vi "Teleop_System_Acquire_Decide.vi"(8 "error in (no error)":errorcluster) -> (0 "error out":errorcluster)   [LabVIEW 2019]
uses:
  <vilib>/Rock Robotics/WPI/Joystick/WPI_JoystickArcadeMapping.vi
  <vilib>/Rock Robotics/WPI/ThirdParty/JAS_Junk/TrajLib/Trajectory_Library.lvlib
  Teleop_System_Globals.vi
  <vilib>/Rock Robotics/WPI/Joystick/XBox Buttons Indexer.ctl
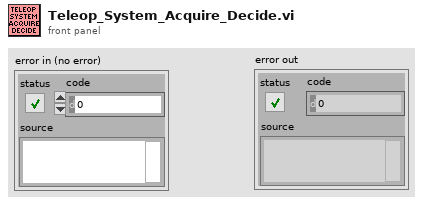
[diagram p1: front panel]
types:
  T1 = typedef "XBox Buttons Indexer.ctl" = enum16{"A", "B", "X", "Y", "Left Bumper", "Right Bumper", "Back", "Start", "Left Joystick", "Right Joystick"}
  T2 = typedef "WPI_JoystickDevRef.ctl" = cluster{"Device":T3}
  T3 = typedef "WPI_JoystickDeviceEnum.ctl" = enum16{"USB 0", "USB 1", "USB 2", "USB 3", "USB 4", "USB 5"}
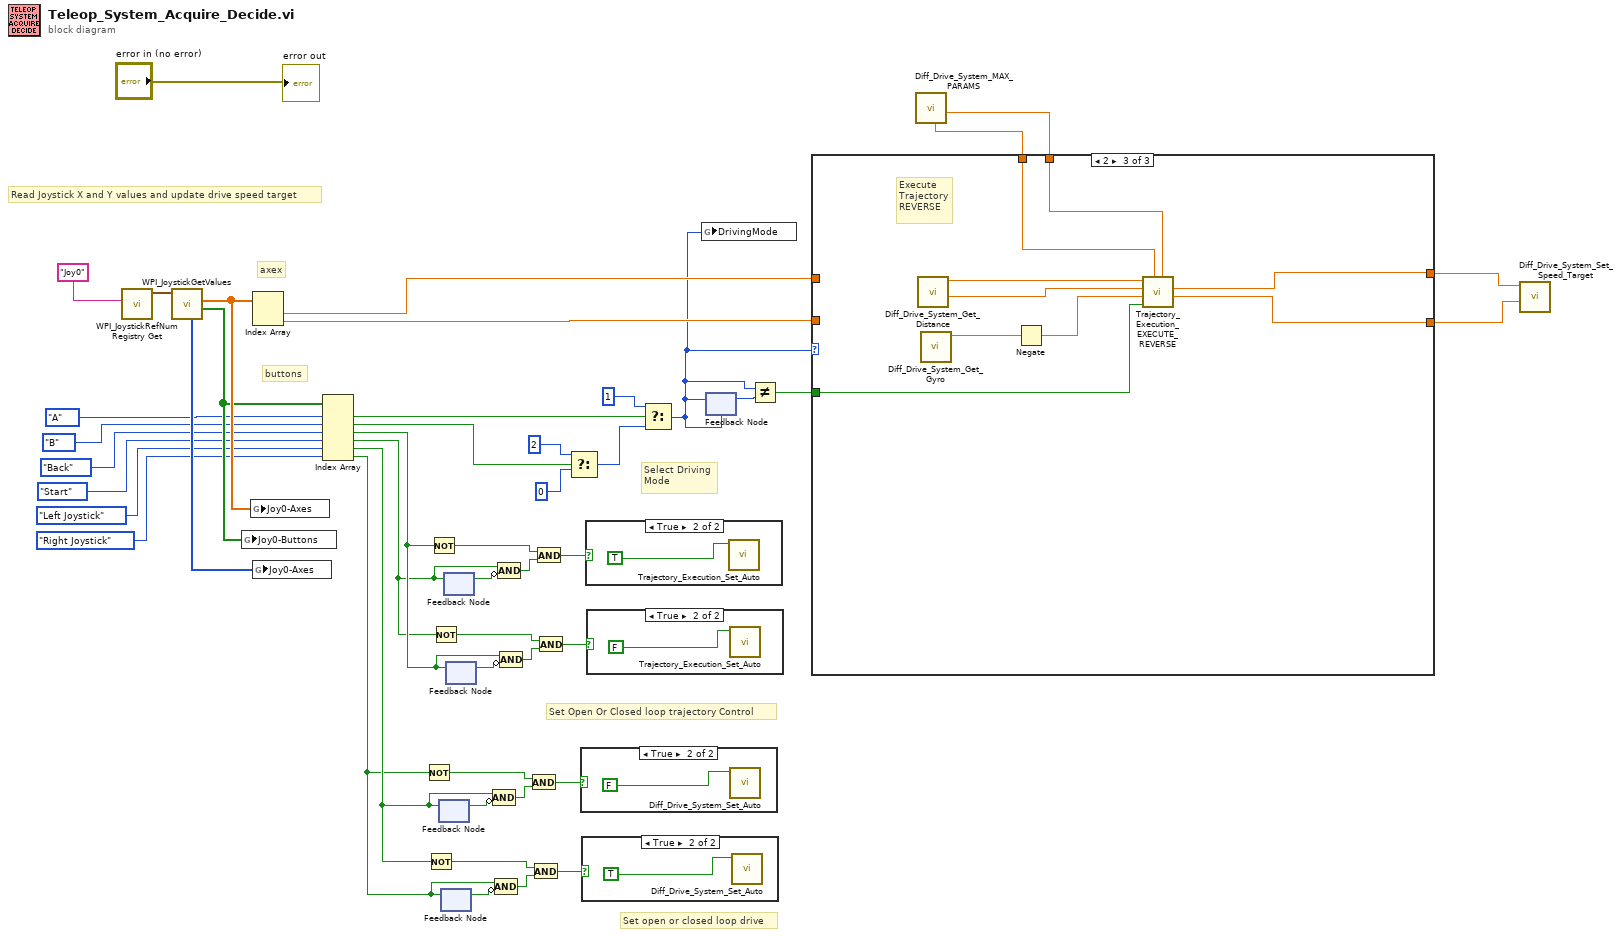
[diagram p0: block diagram]
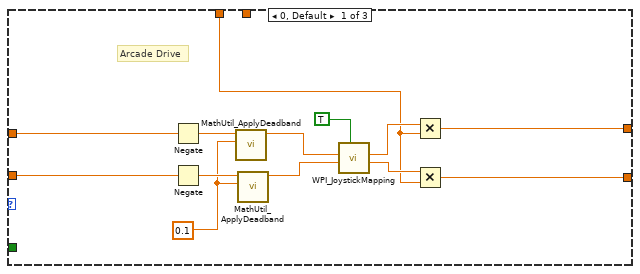
[diagram p6: hidden frame]
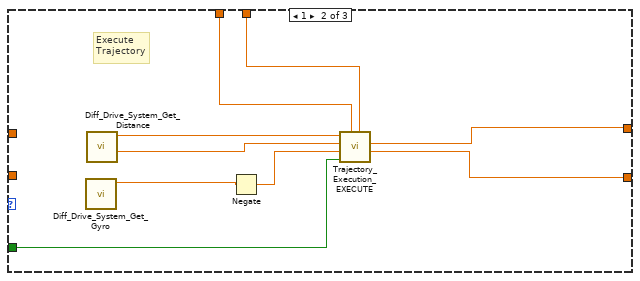
[diagram p7: hidden frame]
diagram:
  # "Set open or closed loop drive"
  # "Set Open Or Closed loop trajectory Control"
  # "Select Driving\nMode"
  # "buttons"
  # "axex"
  # "Read Joystick X and Y values and update drive speed target"
  n1 = call <vilib>:"WPI_JoystickRefNum Registry Get.vi"("refnum name"="Joy0") -> ("JoystickDevRef"=w28:T2)  [unwired: 1 in, 9 out]
  n2 = call <vilib>:"WPI_JoystickGetValues.vi"("JoystickDevRef"=w28) -> ("Buttons"=w25:bool[], "Axes"=w26:dbl[], "POVs"=w24:i16[])  [unwired: 6 in, 2 out]
  n3 = global write "Teleop_System_Globals.vi" "Joy0-Buttons"(w25) -> ()
  n4 = global write "Teleop_System_Globals.vi" "Joy0-Axes"(w26) -> ()
  n5 = Index Array(array=w26) -> (element #1=w29:dbl, element #2=w30:dbl)  [unwired: 2 in]
  n6 = global write "Teleop_System_Globals.vi" "Joy0-Axes"(w24) -> ()
  n7 = Index Array(array=w25, index #1=XBox_Buttons_Indexer."A" ("XBox Buttons"), index #2=XBox_Buttons_Indexer."B" ("XBox Buttons"), index #3=XBox_Buttons_Indexer."Back" ("XBox Buttons"), index #4=XBox_Buttons_Indexer."Start" ("XBox Buttons"), index #5=XBox_Buttons_Indexer."Left Joystick" ("XBox Buttons"), index #6=XBox_Buttons_Indexer."Right Joystick" ("XBox Buttons")) -> (element #1=w32:bool, element #2=w38:bool, element #3=w9:bool, element #4=w8:bool, element #5=w3:bool, element #6=w2:bool)
  n8 = Not(x=w2) -> (.not. x?=w14:bool)
  n9 = Not(x=w3) -> (.not. x?=w17:bool)
  n10 = Not(x=w9) -> (.not. x?=w42:bool)
  n11 = Not(x=w8) -> (.not. x?=w45:bool)
  n12 = feedback #1() -> (w12:bool)  [unwired: 1 in]
  n13 = feedback-in #1(w3) -> ()
  n14 = feedback #2() -> (w15:bool)  [unwired: 1 in]
  n15 = feedback-in #2(w2) -> ()
  n16 = feedback #3() -> (w40:bool)  [unwired: 1 in]
  n17 = feedback-in #3(w8) -> ()
  n18 = feedback #4() -> (w43:bool)  [unwired: 1 in]
  n19 = feedback-in #4(w9) -> ()
  n20 = Compound Arithmetic op=AND(w3, invert w12) -> (w13:bool)
  n21 = Compound Arithmetic op=AND(w2, invert w15) -> (w16:bool)
  n22 = Compound Arithmetic op=AND(w8, invert w40) -> (w41:bool)
  n23 = Compound Arithmetic op=AND(w9, invert w43) -> (w44:bool)
  n24 = And(x=w14, y=w13) -> (x .and. y?=w19:bool)
  n25 = And(x=w17, y=w16) -> (x .and. y?=w18:bool)
  n26 = And(x=w42, y=w41) -> (x .and. y?=w47:bool)
  n27 = And(x=w45, y=w44) -> (x .and. y?=w46:bool)
  n28 = Select(t=2, s=w38, f=0) -> (s? t:f=w37:i32)
  n29 = case shown="True" w19 {
    frame False {
    }
    frame True {
      n30 = call "Diff_Drive_System_Set_Auto.vi"("Auto Mode"=FALSE ("Traj_RamseteEnabled")) -> ()  [unwired: 11 in]
    }
  }
  n31 = case shown="True" w18 {
    frame False {
    }
    frame True {
      n32 = call "Diff_Drive_System_Set_Auto.vi"("Auto Mode"=TRUE ("Traj_RamseteEnabled")) -> ()  [unwired: 11 in]
    }
  }
  n33 = case shown="True" w47 {
    frame False {
    }
    frame True {
      n34 = call "Trajectory_Execution_Set_Auto.vi"("Ramsete AUTO"=TRUE ("Traj_RamseteEnabled")) -> ()  [unwired: 11 in]
    }
  }
  n35 = case shown="True" w46 {
    frame False {
    }
    frame True {
      n36 = call "Trajectory_Execution_Set_Auto.vi"("Ramsete AUTO"=FALSE ("Traj_RamseteEnabled")) -> ()  [unwired: 11 in]
    }
  }
  n37 = Select(t=1, s=w32, f=w37) -> (s? t:f=w20:i32)
  n38 = global write "Teleop_System_Globals.vi" "DrivingMode"(w20) -> ()
  n39 = feedback #5(w20) -> (w33:i32)
  n40 = feedback-in #5(w20) -> ()
  n41 = Not Equal?(x=w20, y=w33) -> (x != y?=w34:bool)
  n42 = call "Diff_Drive_System_MAX_PARAMS.vi"() -> ("Effective TrackWidth Ft"=w39:dbl, "Max Drive Speed Ft/Sec"=w1:dbl)  [unwired: 9 in, 1 out]
  n43 = case shown="2" w20 {
    tunnel: w29 -> [w63 _ _]
    tunnel: w30 -> [w62 _ _]
    tunnel: [w61 w70 w79] -> w22
    tunnel: [w60 w69 w78] -> w21
    tunnel: w1 -> [w57 w71 w80]
    tunnel: w34 -> [_ w73 w82]
    tunnel: w39 -> [_ w68 w77]
    frame 0, Default {
      w52 = 0.1 ("Deadband")
      # "Arcade Drive"
      n44 = Negate(x=w63) -> (-x=w55:dbl)
      n45 = Negate(x=w62) -> (-x=w54:dbl)
      n46 = call <vilib>:"MathUtil_ApplyDeadband.vi"("Deadband"=w52, "Value"=w55) -> ("Result"=w56:dbl)  [unwired: 9 in]
      n47 = call <vilib>:"MathUtil_ApplyDeadband.vi"("Deadband"=w52, "Value"=w54) -> ("Result"=w53:dbl)  [unwired: 9 in]
      n48 = call-poly <vilib>:"WPI_JoystickMapping.vi"("Square Inputs"=TRUE, "Y axis value"=w53, "X axis value"=w56) -> ("Right Motor Value"=w58:dbl, "Left Motor Value"=w59:dbl)  [unwired: 7 in]
      n49 = Multiply(x=w59, y=w57) -> (x*y=w61:dbl)
      n50 = Multiply(x=w58, y=w57) -> (x*y=w60:dbl)
    }
    frame 1 {
      # "Execute\nTrajectory"
      n51 = call "Diff_Drive_System_Get_Gyro.vi"() -> ("Gyro_DEG"=w67:dbl)  [unwired: 10 in, 1 out]
      n52 = call "Diff_Drive_System_Get_Distance.vi"() -> ("Right Distance FT"=w65:dbl, "Left Distance FT"=w66:dbl)  [unwired: 10 in]
      n53 = Negate(x=w67) -> (-x=w72:dbl)
      n54 = call "Trajectory_Execution_EXECUTE.vi"("Track Width FT"=w68, "Max Speed\nFT/SEC"=w71, "Init"=w73, "Gyro Continous\n (inc counterclockwise)"=w72, "Right Distance"=w65, "Left Distance"=w66) -> ("Right Speed Target"=w69:dbl, "Left Speed Target"=w70:dbl)  [unwired: 1 in, 3 out]
    }
    frame 2 {
      # "Execute\nTrajectory\nREVERSE"
      n55 = call "Diff_Drive_System_Get_Distance.vi"() -> ("Right Distance FT"=w74:dbl, "Left Distance FT"=w75:dbl)  [unwired: 10 in]
      n56 = call "Diff_Drive_System_Get_Gyro.vi"() -> ("Gyro_DEG"=w76:dbl)  [unwired: 10 in, 1 out]
      n57 = Negate(x=w76) -> (-x=w81:dbl)
      n58 = call "Trajectory_Execution_EXECUTE_REVERSE.vi"("Track Width FT"=w77, "Max Speed\nFT/SEC"=w80, "Init"=w82, "Gyro Continous\n (inc counterclockwise)"=w81, "Right Distance"=w74, "Left Distance"=w75) -> ("Right Speed Target"=w78:dbl, "Left Speed Target"=w79:dbl)  [unwired: 1 in, 3 out]
    }
  }
  n59 = call "Diff_Drive_System_Set_Speed_Target.vi"("Right Speed Target FT/S"=w21, "Left Speed Target FT/S"=w22) -> ()  [unwired: 10 in]
  "error out" <- "error in (no error)"
